vi "String Array to Logcluster Array.vi"(8 "error in (no error)":errorcluster, 11 "LogString Array":string[](array[string])) -> (0 "error out":errorcluster, 3 "Array":T1[](array[typedef]))   [LabVIEW 2012]
uses:
  typedef/Log_User_Data.ctl
  typedef/User Accounts.ctl
panel:
  in  "Array 2":T1[](array[typedef])
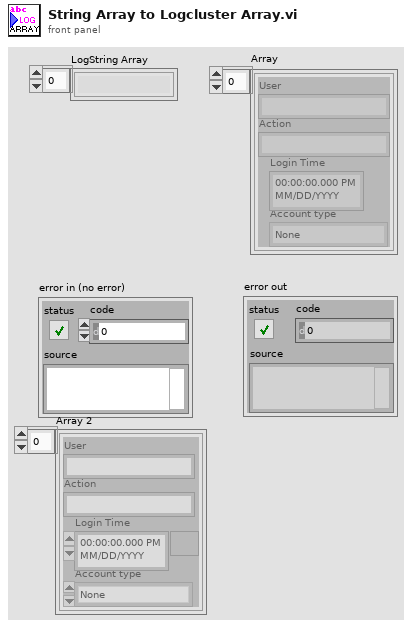
[diagram p1: front panel]
types:
  T1 = typedef "Log_User_Data.ctl" = cluster{"User":string, "Action":string, "Account type":T2, "Login Time ":timestamp}
  T2 = typedef "User Accounts.ctl" = enum16{"None", "User", "Admin"}
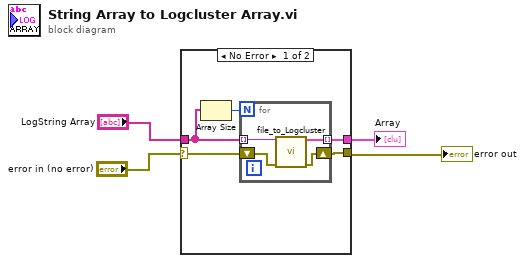
[diagram p0: block diagram]
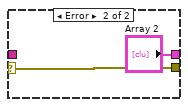
[diagram p2: hidden frame]
diagram:
  n1 = case shown="No Error" "error in (no error)" {
    selector: "error in (no error)" -> [w5 w14]
    tunnel: "LogString Array" -> [w9 _]
    tunnel: [w8 "Array 2"] -> w3
    tunnel: [w6 w14] -> w1
    frame No Error {
      n2 = Array Size(array=w9) -> (size(s)=w7:i32)
      n3 = for {
        N: w7 -> [_]
        tunnel: [w12] -> w8 mode=indexing
        tunnel: w9 -> [w13] mode=indexing
        shift-right: [w11] -> w6
        shift-left: w5 -> [w10]
        n4 = call "file_to_Logcluster.vi"("Cyphered text"=w13, "error in (no error)"=w10) -> ("Log Cluster Out"=w12:T1, "error out"=w11:errorcluster)  [unwired: 12 in]
      }
    }
    frame Error {
    }
  }
  "Array" <- w3
  "error out" <- w1
